vi "Split String.vi"(2 "String":string, 4 "Delimiter":string) -> (7 "Elements":string[](array[string]))   [LabVIEW 2017, in "Request.lvclass"]
uses:
  Request.lvclass
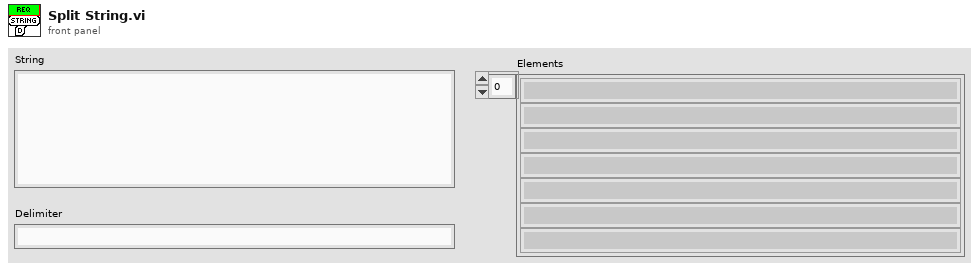
[diagram p1: front panel]
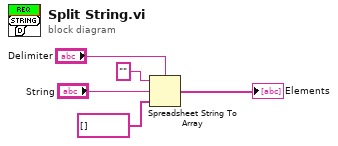
[diagram p0: block diagram]
diagram:
  n1 = Spreadsheet String To Array(delimiter (Tab)="Delimiter", format string="", spreadsheet string="String", array type (2D Dbl)=string[] []) -> (array=→"Elements":string[])
